vi "DVR.baseFolder.Write.vi"(8 "error in":errorcluster, 10 "save.base_folder":cluster{"Folder":path, "tif":bool, "jpg":bool}, 11 "DVR in":T1) -> (0 "error out":errorcluster)   [LabVIEW 2020]
uses:
  _controls/data.ctl
  camera/camera.lvclass
  _controls/data.ref.ctl
  <vilib>/vision/Image Controls.llb/IMAQ Image.ctl
  _controls/state.ctl
  _controls/data.vars.ctl
  _controls/flip.ctl
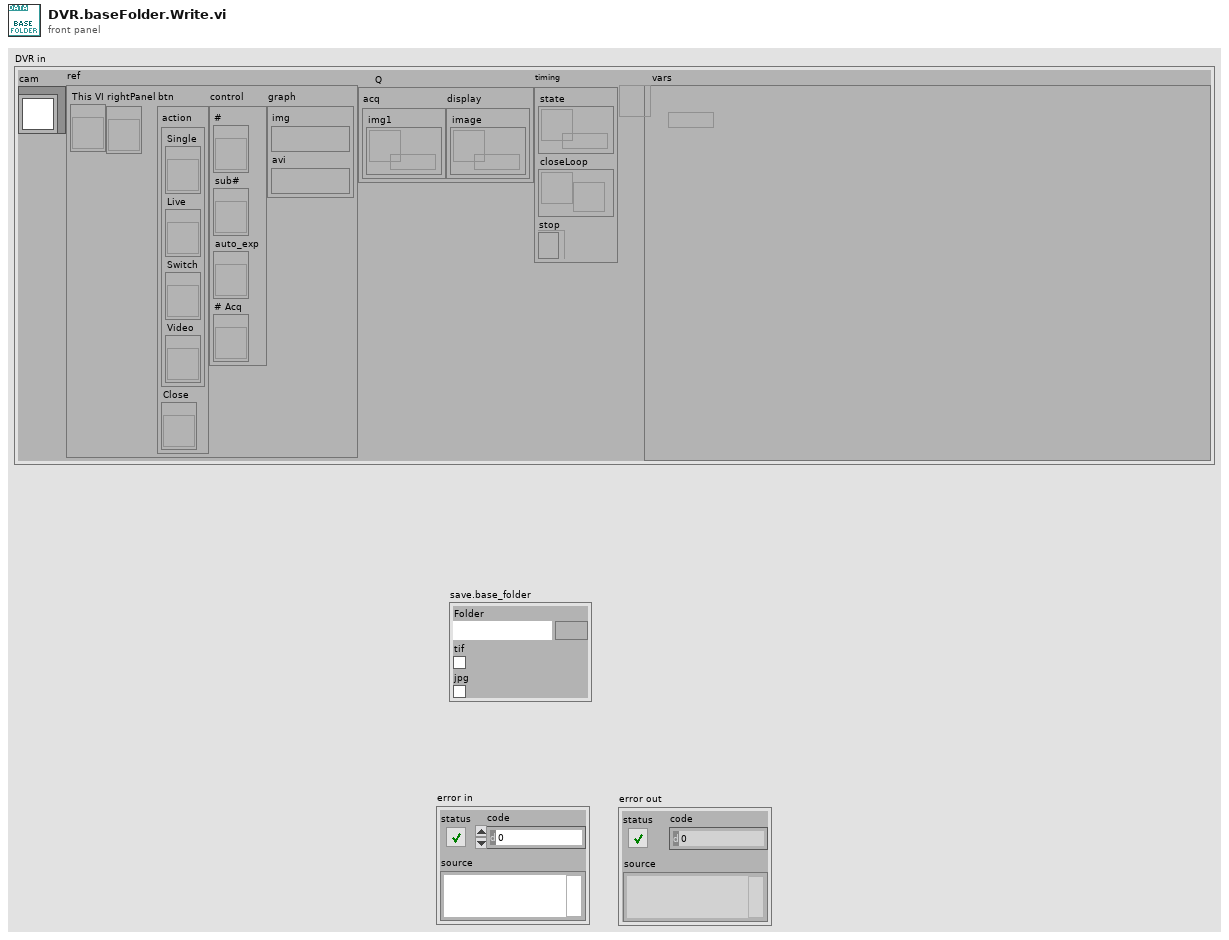
[diagram p1: front panel]
types:
  T1 = typedef "data.ctl" = cluster{"cam":refnum<class "camera.lvclass">, "ref":T2, "Q":cluster{"acq":cluster{"img1":refnum<queue>}, "display":cluster{"image":refnum<queue>}}, "timing":cluster{"state":refnum<queue>, "closeLoop":refnum<notifier>, "stop":refnum<k4>}, "vars":refnum<data-value>}
  T2 = typedef "data.ref.ctl" = cluster{"This VI":refnum<vi>, "rightPanel":refnum<vi>, "btn":cluster{"action":cluster{"Single":refnum<vi>, "Live":refnum<vi>, "Switch":refnum<vi>, "Video":refnum<vi>}, "Close":refnum<vi>}, "control":cluster{"#":refnum<vi>, "sub#":refnum<vi>, "auto_exp":refnum<vi>, "# Acq":refnum<vi>}, "graph":cluster{"img":T3, "avi":T3}}
  T3 = typedef "IMAQ Image.ctl" = refnum<image>
  T4 = typedef "data.vars.ctl" = cluster{"save":cluster{"base_folder":cluster{"Folder":path, "tif":bool, "jpg":bool}, "module":string, "#":u32, "sub#":u8, "save.op":enum16{"Full", "Light"}, "same?":bool, "Shift":enum16{"Single", "Leapfrog"}, "jpg?":bool, "flip":T5}, "acq":cluster{"# Acq":u16, "rotate":bool, "FPS":dbl}, "calib.manual":cluster{"BG":cluster{"Image":u16[][], "enabled?":bool}, "FF":cluster{"Image":u16[][], "enabled?":bool}}}
  T5 = typedef "flip.ctl" = cluster{"x":bool, "y":bool}
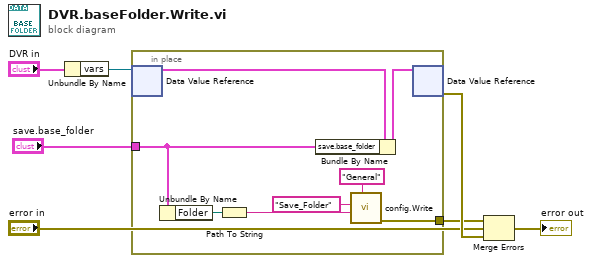
[diagram p0: block diagram]
diagram:
  n1 = Unbundle By Name("DVR in") -> ("vars"=w6:refnum<data-value>)
  n2 = in-place {
    in-place-border: [w13] -> w2
    in-place-border: "save.base_folder" -> [w9]
    n3 = in-place-dvr #1(w6) -> (w15:T4)  [unwired: 1 out]
    n4 = Unbundle By Name(w9) -> ("Folder"=w8:path)
    n5 = Path To String(path=w8) -> (string=w11:string)
    n6 = Bundle By Name(cluster=w15, "save.base_folder"=w9) -> (w14:T4)
    n7 = call "config.Write.vi"("section"="General", "value"=w11, "key"="Save_Folder") -> ("error out"=w13:errorcluster)  [unwired: 8 in]
    n8 = in-place-dvr #1(w14) -> (w7:errorcluster)  [unwired: 1 out]
  }
  n9 = Merge Errors(w2, "error in", w7) -> (→"error out":errorcluster)
